vi "createQueueTcpClientFromDds.vi"(8 "error in (no error)":errorcluster, 11 "tcpServerTel in":refnum<class "TcpServerTel.lvclass">) -> (0 "error out":errorcluster, 3 "tcpServerTel out":refnum<class "TcpServerTel.lvclass">)   [LabVIEW 2018, in "TcpServerTel.lvclass"]
doc: "Create telemetry queue to pass packets from TCP Server to LabVIEW Component."
uses:
  TcpServerTel.lvclass
  TcpServerTel.lvclass/TcpServerTel.ctl
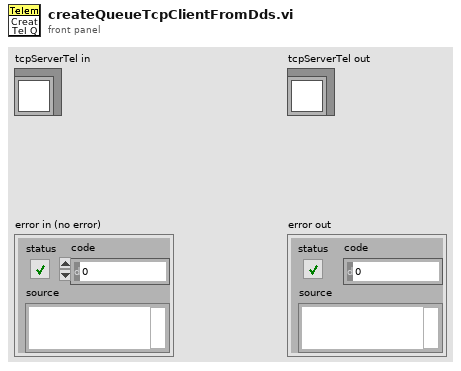
[diagram p1: front panel]
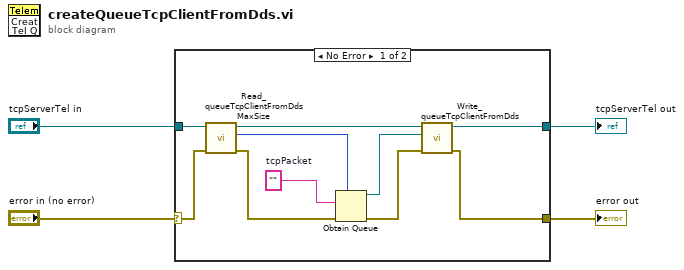
[diagram p0: block diagram]
diagram:
  n1 = case shown="No Error" "error in (no error)" {
    selector: "error in (no error)" -> [w5 w16]
    tunnel: "tcpServerTel in" -> [w14 w15]
    tunnel: [w13 w15] -> w3
    tunnel: [w9 w16] -> w1
    frame No Error {
      w11 = ""  # tcpPacket
      n2 = call "Read_queueTcpClientFromDdsMaxSize.vi"("error in (no error)"=w5, "TcpServerTel in"=w14) -> ("error out"=w6:errorcluster, "queueTcpClientFromDdsMaxSize"=w7:i32, "TcpServerTel out"=w8:refnum<class "TcpServerTel.lvclass">)  [unwired: 7 in]
      n3 = Obtain Queue(max queue size (-1, unlimited)=w7, element data type=w11, error in (no error)=w6) -> (queue out=w10:refnum<queue>, error out=w12:errorcluster)  [unwired: 2 in, 1 out]
      n4 = call "Write_queueTcpClientFromDds.vi"("error in (no error)"=w12, "queueTcpClientFromDds"=w10, "TcpServerTel in"=w8) -> ("error out"=w9:errorcluster, "TcpServerTel out"=w13:refnum<class "TcpServerTel.lvclass">)  [unwired: 7 in]
    }
    frame Error {
    }
  }
  "error out" <- w1
  "tcpServerTel out" <- w3
